vi "calibrate all.vi"(4 "Calibration parameters":T6={"Calibrated output"=0.0, "2nd channel"=[], "2nd Channel Index"=0, "Dissolved Oxygen"={"Temperature Index"=0, "Temperature (C)"=20.0, "Temperature\ncompensation"=FALSE, "Barometric Pressure (kPa)"=101.3}, "pH"={"Buffers"=[4.0, 7.0, 10.0], "Temperature \ncompensation"=FALSE, "Temperature Index"=0, "Temperature (C)"=20.0}, "Channel Name"=[]} {"pH"."Temperature (C)" format="%.2f"; "pH"."Buffers" format="%.2f"; "Dissolved Oxygen"."Barometric Pressure (kPa)" format="%.2f"; "Dissolved Oxygen"."Temperature (C)" format="%.2f"; "Calibrated output" format="%.2f"}, 5 "Connection ID":refnum<k5>, 10 "Index":u32, 11 "Ports":T7) -> ()   [LabVIEW 2010]
uses:
  DAQ configuration/Sensor buffer command.ctl
  DAQ configuration/channel identifier.ctl
  DAQ configuration/Sensor array.ctl
  Dissolved Oxygen/DO.ctl
  calibration parameters.ctl
  pH/pH calibration.ctl
  DAQ configuration/scale type.ctl
  correspondence table.ctl
  pH/pH scale.ctl
  Dissolved Oxygen/DO scale.ctl
  conversion.ctl
panel:
  out "Conversion Array out":T1[](array[typedef]) {"D.O."."K" format="%.6f"; "D.O."."Temperature" format="%.2f"; "pH scale"."Buffers"."V/T" format="%.5f"; "pH scale"."Buffers"."Buffer" format="%.2f"; "pH scale"."Temperature" format="%.2f"; "offset (physical units)" format="%.5f"; "correspondence table"."volts" format="%.4f"; "correspondence table"."physical units" format="%.4f"; "second channel" min=-1; "offset (volts)" format="%.5f"; "conversion matrix" format="%.4e"}
  in  "Conversion Array":T1[](array[typedef]) {"D.O."."K" format="%.6f"; "D.O."."Temperature" format="%.2f"; "pH scale"."Buffers"."V/T" format="%.5f"; "pH scale"."Buffers"."Buffer" format="%.2f"; "pH scale"."Temperature" format="%.2f"; "offset (physical units)" format="%.5f"; "correspondence table"."volts" format="%.4f"; "correspondence table"."physical units" format="%.4f"; "second channel" min=-1; "offset (volts)" format="%.5f"; "conversion matrix" format="%.4e"}
  # "C"
  # "kPa"
  # "C"
  # "C"
  # "kPa"
  # "C"
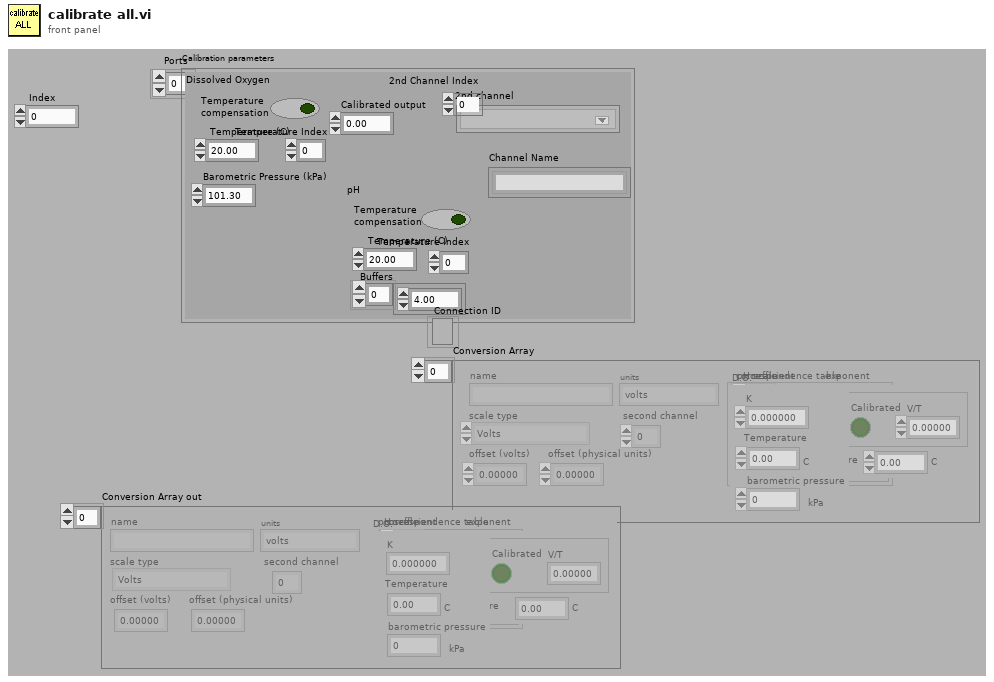
[diagram p1: front panel]
types:
  T1 = typedef "conversion.ctl" = cluster{"conversion matrix":sgl[][], "units":string, "name":string, "scale type":T2, "offset (volts)":dbl, "second channel":i8, "correspondence table":T3, "offset (physical units)":dbl, "pH scale":T4, "D.O.":T5}
  T2 = typedef "scale type.ctl" = enum16{"Volts", "Polynomial", "Correspondence Table", "pH", "Dissolved Oxygen", "Quadratic"}
  T3 = typedef "correspondence table.ctl" = cluster{"physical units":dbl, "volts":dbl}[]
  T4 = typedef "pH scale.ctl" = cluster{"Buffers":cluster{"Buffer":dbl, "Calibrated":bool, "V/T":dbl}[], "Temperature":dbl}
  T5 = typedef "DO scale.ctl" = cluster{"Temperature":dbl, "K":dbl, "barometric pressure":dbl}
  T6 = typedef "calibration parameters.ctl" = cluster{"Calibrated output":dbl, "2nd channel":T7, "2nd Channel Index":u32, "Dissolved Oxygen":T9, "pH":T10, "Channel Name":string[]}
  T7 = typedef "Sensor array.ctl" = T8[]
  T8 = typedef "channel identifier.ctl" = u16
  T9 = typedef "DO.ctl" = cluster{"Temperature Index":u32, "Temperature (C)":dbl, "Temperature\ncompensation":bool, "Barometric Pressure (kPa)":dbl}
  T10 = typedef "pH calibration.ctl" = cluster{"Buffers":dbl[], "Temperature \ncompensation":bool, "Temperature Index":u32, "Temperature (C)":dbl}
  T11 = cluster{"Buffers":cluster{"Buffer":dbl, "Calibrated":bool, "V/T":dbl}[], "Temperature":dbl}
  T12 = enum16{"Volts", "Polynomial", "Correspondence Table", "pH", "Dissolved Oxygen"}
  T13 = typedef "Sensor buffer command.ctl" = enum16{"read average", "read recent", "read all", "write", "configure", "clear"}
  T14 = enum16{"Volts", "Polynomial", "Correspondence Table", "pH", "Dissolved Oxygen", "Quadratic"}
  T15 = typedef "Sensor data.ctl" = cluster{" Sensor array":T16[], "Time":dbl}
  T16 = typedef "sensor cluster.ctl" = cluster{"voltage":sgl, "scaled":sgl, "units":string, "Out of Range":bool}
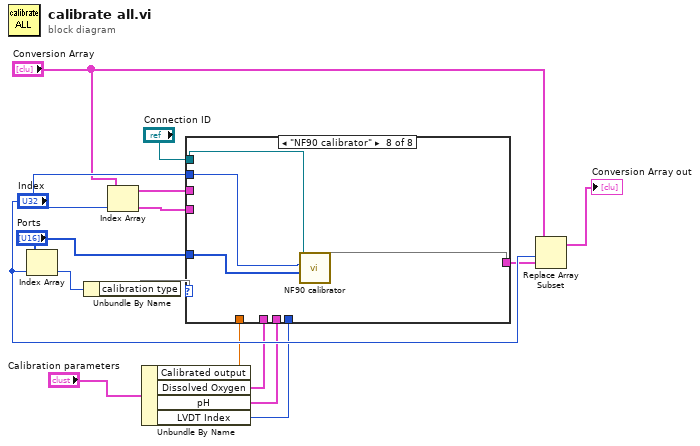
[diagram p0: block diagram]
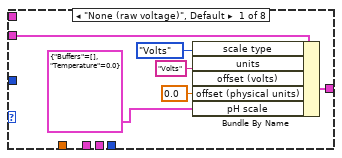
[diagram p2: hidden frame]
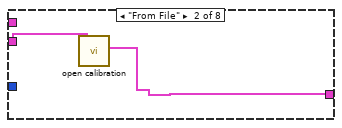
[diagram p3: hidden frame]
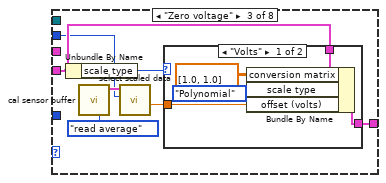
[diagram p4: hidden frame]
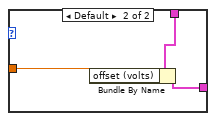
[diagram p5: hidden frame]
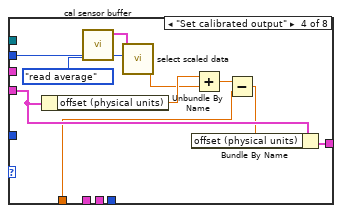
[diagram p6: hidden frame]
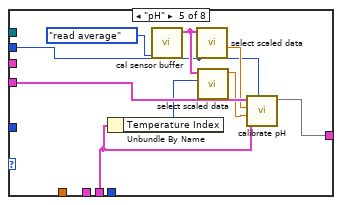
[diagram p7: hidden frame]
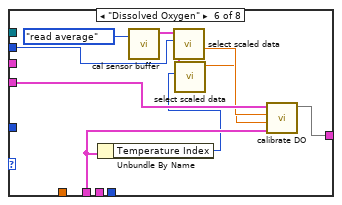
[diagram p8: hidden frame]
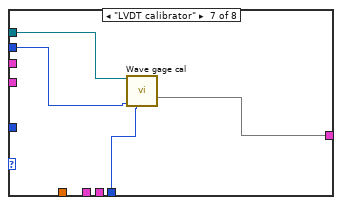
[diagram p9: hidden frame]
diagram:
  n1 = Index Array(array="Ports", index="Index") -> (element=w10:T8)
  n2 = Unbundle By Name(w10) -> ("calibration type"=w9)
  n3 = Index Array(array="Conversion Array", index="Index") -> (element=w14:T1)
  n4 = Unbundle By Name("Calibration parameters") -> ("Calibrated output"=w6:dbl, "Dissolved Oxygen"=w7:T9, "pH"=w3:T10, "LVDT Index"=w4:u32)
  n5 = case shown="\"NF90 calibrator\"" w9 {
    tunnel: w14 -> [w18 w22 w28 w47 w55 w65 _ _]
    tunnel: [w17 w21 w27 w46 w56 w64 w68 w73] -> w12
    tunnel: "Index" -> [_ _ w25 w39 w48 w62 w69 w72]
    tunnel: "Ports" -> [_ _ _ _ _ _ _ w70]
    tunnel: w7 -> [_ _ _ _ _ w61 _ _]
    tunnel: w6 -> [_ _ _ w42 _ _ _ _]
    tunnel: "Connection ID" -> [_ _ _ _ _ _ w67 w71]
    tunnel: "Conversion Array" -> [_ _ _ _ _ _ _ _]
    tunnel: w4 -> [_ _ _ _ _ _ w66 _]
    tunnel: w3 -> [_ _ _ _ w52 _ _ _]
    frame "None (raw voltage)", Default {
      w16 = 0.0 ("offset (volts)")
      n6 = Bundle By Name(cluster=w18, "scale type"=T12."Volts", "units"="Volts", "offset (volts)"=w16, "offset (physical units)"=w16, "pH scale"=T11 {"Buffers"=[], "Temperature"=0.0}) -> (w17:T1)
    }
    frame "From File" {
      n7 = call "open calibration.vi"(6:w22) -> ("conversion out"=w21:T1)  [unwired: 6 in]
    }
    frame "Zero voltage" {
      n8 = Unbundle By Name(w28) -> ("scale type"=w29:T2)
      n9 = call "cal sensor buffer.vi"("command"=Sensor_buffer_command."read average") -> ("Sensor Data smoothed"=w26:T15)  [unwired: 4 in, 2 out]
      n10 = call "select scaled data.vi"("Sensor index"=w25, "Sensor Data"=w26) -> ("voltage"=w23:sgl)  [unwired: 3 in, 4 out]
      n11 = case shown="\"Volts\"" w29 {
        tunnel: w28 -> [w34 w37]
        tunnel: w23 -> [w32 w35]
        tunnel: [w30 w36] -> w27
        frame "Volts" {
          n12 = Bundle By Name(cluster=w34, "conversion matrix"=sgl[][] [[1.0, 1.0]], "scale type"=T14."Polynomial", "offset (volts)"=w32) -> (w30:T1)
        }
        frame Default {
          n13 = Bundle By Name(cluster=w37, "offset (volts)"=w35) -> (w36:T1)
        }
      }
    }
    frame "Set calibrated output" {
      n14 = Unbundle By Name(w47) -> ("offset (physical units)"=w45:dbl)
      n15 = call "cal sensor buffer.vi"("command"=Sensor_buffer_command."read average") -> ("Sensor Data smoothed"=w40:T15)  [unwired: 4 in, 2 out]
      n16 = call "select scaled data.vi"("Sensor index"=w39, "Sensor Data"=w40) -> ("scaled"=w38:sgl)  [unwired: 3 in, 4 out]
      n17 = Add(x=w45, y=w38) -> (x+y=w44:dbl)
      n18 = Subtract(x=w44, y=w42) -> (x-y=w43:dbl)
      n19 = Bundle By Name(cluster=w47, "offset (physical units)"=w43) -> (w46:T1)
    }
    frame "pH" {
      n20 = Unbundle By Name(w52) -> ("Temperature Index"=w51:u32)
      n21 = call "cal sensor buffer.vi"("command"=Sensor_buffer_command."read average") -> ("Sensor Data smoothed"=w53:T15)  [unwired: 4 in, 2 out]
      n22 = call "select scaled data.vi"("Sensor index"=w48, "Sensor Data"=w53) -> ("voltage"=w50:sgl)  [unwired: 3 in, 4 out]
      n23 = call "select scaled data.vi"("Sensor index"=w51, "Sensor Data"=w53) -> ("scaled"=w49:sgl)  [unwired: 3 in, 4 out]
      n24 = call "calibrate pH.vi"("index"=w48, "pH"=w52, "Temperature"=w49, "pH voltage"=w50, 11:w55) -> (3:w56)  [unwired: 6 in]
    }
    frame "Dissolved Oxygen" {
      n25 = Unbundle By Name(w61) -> ("Temperature Index"=w60:u32)
      n26 = call "cal sensor buffer.vi"("command"=Sensor_buffer_command."read average") -> ("Sensor Data smoothed"=w59:T15)  [unwired: 4 in, 2 out]
      n27 = call "select scaled data.vi"("Sensor index"=w62, "Sensor Data"=w59) -> ("voltage"=w58:sgl)  [unwired: 3 in, 4 out]
      n28 = call "select scaled data.vi"("Sensor index"=w60, "Sensor Data"=w59) -> ("scaled"=w57:sgl)  [unwired: 3 in, 4 out]
      n29 = call "calibrate DO.vi"(8:w61, 9:w57, 10:w58, "Index"=w65) -> (3:w64)  [unwired: 7 in]
    }
    frame "LVDT calibrator" {
      n30 = call "Wave gage cal.vi"("refnum in"=w67, "Uncalibrated index"=w69, "Reference Index"=w66) -> (10:w68)  [unwired: 12 in]
    }
    frame "NF90 calibrator" {
      n31 = call "NF90 calibrator.vi"("Ports"=w70, "channel index"=w72, "data server address"=w71) -> (3:w73)  [unwired: 8 in]
    }
  }
  n32 = Replace Array Subset(array="Conversion Array", new element=w12, index="Index") -> (→"Conversion Array out":T1[])
